vi "Update All Values.vi"(8 "error in (no error)":errorcluster, 10 "Values":refnum<class "Type.lvclass">[](array[class]), 11 "User in":refnum<class "User.lvclass">) -> (0 "error out":errorcluster, 3 "User out":refnum<class "User.lvclass">)   [LabVIEW 2022 SP3, in "Conditum-Example.lvlib" / "User.lvclass"]
uses:
  User.lvclass
  Conditum/Columns/Type/Type.lvclass
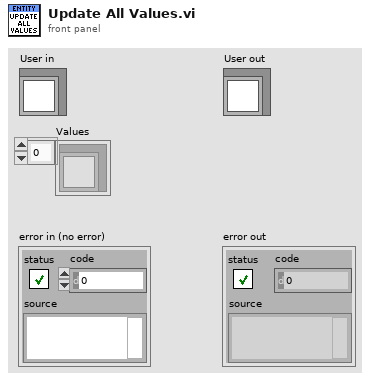
[diagram p1: front panel]
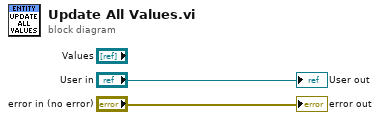
[diagram p0: block diagram]
diagram:
  "error out" <- "error in (no error)"
  "User out" <- "User in"
